vi "Update Test Data Table.vi"(6 "Enum":enum16{"PSU", "Mic"}(ring), 7 "Prev Result in":bool, 8 "Error In":errorcluster, 9 "Test Data In":dbl[](array[numeric]), 10 "Limit In":T1, 11 "Test Data ref in":refnum<vi>) -> (0 "Error Out":errorcluster, 2 "Latest Result Out":bool)   [LabVIEW 2018]
uses:
  Types/LimitType.ctl
panel:
  # "Add PSU Data"
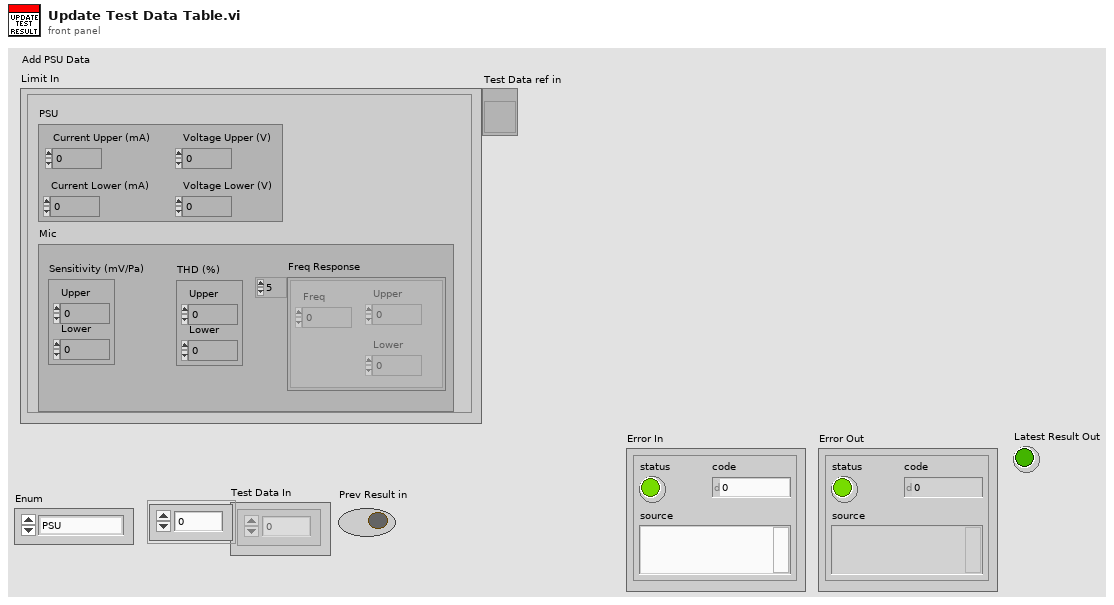
[diagram p1: front panel]
types:
  T1 = typedef "LimitType.ctl" = cluster{"PSU":cluster{"Current Lower (mA)":dbl, "Current Upper (mA)":dbl, "Voltage Lower (V)":dbl, "Voltage Upper (V)":dbl}, "Mic":cluster{"Sensitivity (mV/Pa)":cluster{"Lower":dbl, "Upper":dbl}, "THD (%)":cluster{"Lower":dbl, "Upper":dbl}, "Freq Response":cluster{"Freq":dbl, "Upper":dbl, "Lower":dbl}[]}}
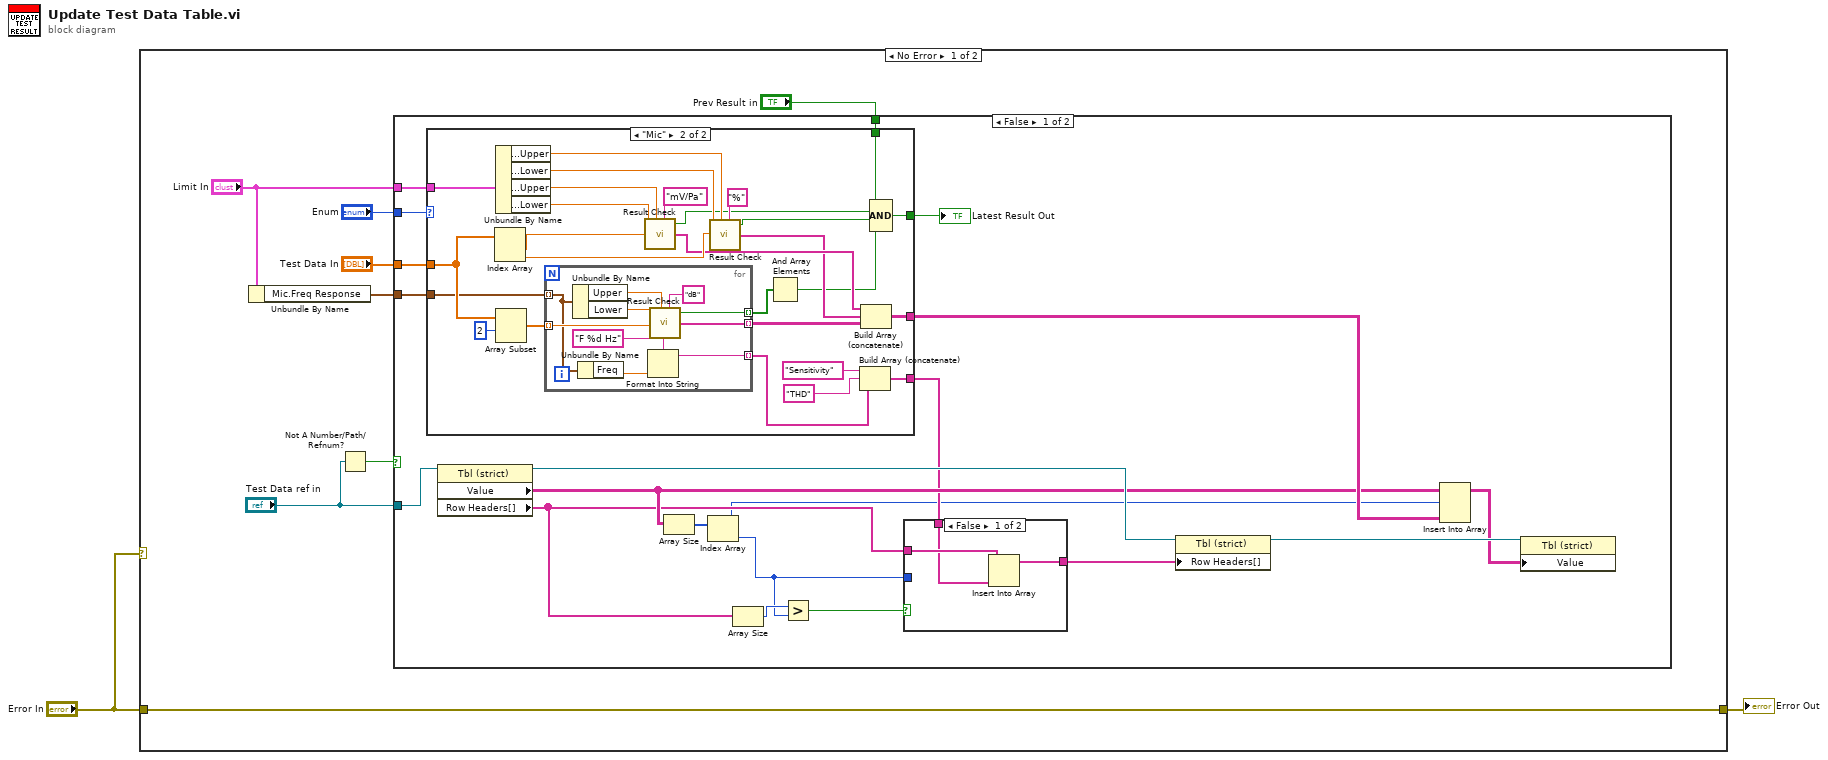
[diagram p0: block diagram]
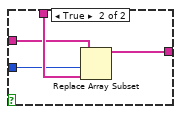
[diagram p2: hidden frame]
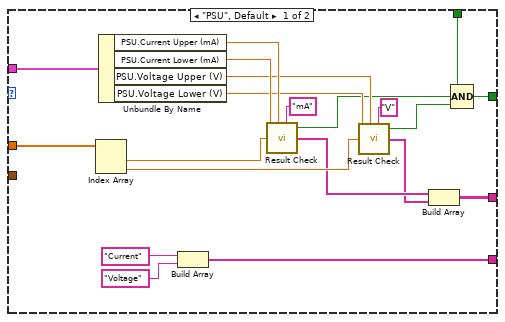
[diagram p3: hidden frame]
diagram:
  n1 = case shown="No Error" "Error In" {
    tunnel: "Error In" -> [w3 w94]
    tunnel: [w3 w94] -> w1
    frame No Error {
      n2 = Unbundle By Name("Limit In") -> ("Mic.Freq Response"=w5:cluster{"Freq":dbl, "Upper":dbl, "Lower":dbl}[])
      n3 = Not A Number/Path/Refnum?(number/path/refnum="Test Data ref in") -> (NaN/Path/Refnum?=w10:bool)
      n4 = case shown="False" w10 {
        tunnel: "Test Data ref in" -> [w29 _]
        tunnel: "Enum" -> [w27 _]
        tunnel: "Limit In" -> [w26 _]
        tunnel: "Test Data In" -> [w25 _]
        tunnel: w5 -> [w17 _]
        tunnel: "Prev Result in" -> [w16 _]
        frame False {
          n5 = case shown="\"Mic\"" w27 {
            tunnel: w26 -> [w56 w83]
            tunnel: w25 -> [w53 w72]
            tunnel: [w46 w63] -> w24
            tunnel: [w41 w67] -> w19
            tunnel: w17 -> [_ w70]
            tunnel: w16 -> [w40 w62]
            tunnel: [w37 w60] -> w15
            frame "PSU", Default {
              n6 = Index Array(array=w53) -> (element #1=w52:dbl, element #2=w49:dbl)  [unwired: 2 in]
              n7 = Unbundle By Name(w56) -> ("PSU.Current Upper (mA)"=w55:dbl, "PSU.Current Lower (mA)"=w54:dbl, "PSU.Voltage Upper (V)"=w51:dbl, "PSU.Voltage Lower (V)"=w50:dbl)
              n8 = Build Array("Current", "Voltage") -> (w41:string[])
              n9 = call "Result Check.vi"("Lower"=w54, "Upper"=w55, "Test Data"=w52, "Unit"="mA") -> ("Result"=w39:bool, "Result String Array Out"=w48:string[])  [unwired: 4 in]
              n10 = call "Result Check.vi"("Lower"=w50, "Upper"=w51, "Test Data"=w49, "Unit"="V") -> ("Result"=w38:bool, "Result String Array Out"=w47:string[])  [unwired: 4 in]
              n11 = Build Array(w48, w47) -> (w46:string[][])
              n12 = Compound Arithmetic op=AND(w40, w39, w38) -> (w37:bool)
            }
            frame "Mic" {
              n13 = Index Array(array=w72) -> (element #1=w77:dbl, element #2=w73:dbl)  [unwired: 2 in]
              n14 = Unbundle By Name(w83) -> ("Mic.THD (%).Upper"=w76:dbl, "Mic.THD (%).Lower"=w75:dbl, "Mic.Sensitivity (mV/Pa).Upper"=w80:dbl, "Mic.Sensitivity (mV/Pa).Lower"=w79:dbl)
              n15 = Array Subset(array=w72, index=2) -> (w69:dbl[])  [unwired: 1 in]
              n16 = for {
                tunnel: w70 -> [w88] mode=indexing
                tunnel: w69 -> [w91] mode=indexing
                tunnel: [w89] -> w64 mode=indexing
                tunnel: [w85] -> w68 mode=indexing
                tunnel: [w84] -> w58 mode=indexing
                n17 = Unbundle By Name(w88) -> ("Upper"=w93:dbl, "Lower"=w92:dbl)
                n18 = Unbundle By Name(w88) -> ("Freq"=w86:dbl)
                n19 = Format Into String(format string="F %d Hz", w86) -> (resulting string=w85:string)  [unwired: 2 in, 1 out]
                n20 = call "Result Check.vi"("Lower"=w92, "Upper"=w93, "Test Data"=w91, "Unit"="dB") -> ("Result"=w84:bool, "Result String Array Out"=w89:string[])  [unwired: 4 in]
              }
              n21 = call "Result Check.vi"("Lower"=w79, "Upper"=w80, "Test Data"=w77, "Unit"="mV/Pa") -> ("Result"=w61:bool, "Result String Array Out"=w66:string[])  [unwired: 4 in]
              n22 = call "Result Check.vi"("Lower"=w75, "Upper"=w76, "Test Data"=w73, "Unit"="%") -> ("Result"=w59:bool, "Result String Array Out"=w65:string[])  [unwired: 4 in]
              n23 = And Array Elements(Boolean array=w58) -> (logical AND=w57:bool)
              n24 = Build Array (concatenate)("Sensitivity", "THD", w68) -> (w67:string[])
              n25 = Build Array (concatenate)(w66, w65, w64) -> (w63:string[][])
              n26 = Compound Arithmetic op=AND(w62, w61, w59, w57) -> (w60:bool)
            }
          }
          "Latest Result Out" <- w15
          n27 = property class="Tbl (strict)"(reference=w29) -> (reference out=w28:refnum<vi>, "Value"=w20:string[][], "Row Headers[]"=w14:string[])  [unwired: 1 in, 1 out]
          n28 = Array Size(array=w20) -> (size(s)=w21:i32[])
          n29 = Index Array(array=w21) -> (element=w11:i32)  [unwired: 1 in]
          n30 = Array Size(array=w14) -> (size(s)=w12:i32)
          n31 = Greater?(x=w12, y=w11) -> (0:w13:bool)
          n32 = case shown="False" w13 {
            tunnel: w19 -> [w31 w36]
            tunnel: [w30 w35] -> w18
            tunnel: w14 -> [w32 w33]
            tunnel: w11 -> [_ w34]
            frame False {
              n33 = Insert Into Array(array=w32, new element=w31) -> (w30:string[])  [unwired: 1 in]
            }
            frame True {
              n34 = Replace Array Subset(array=w33, new element=w36, index=w34) -> (w35:string[])
            }
          }
          n35 = property class="Tbl (strict)"(reference=w28, "Row Headers[]"=w18) -> (reference out=w23:refnum<vi>)  [unwired: 1 in, 1 out]
          n36 = Insert Into Array(array=w20, index (row)=w11, new element=w24) -> (w22:string[][])  [unwired: 1 in]
          n37 = property class="Tbl (strict)"(reference=w23, "Value"=w22) -> ()  [unwired: 1 in, 2 out]
        }
        frame True {
        }
      }
    }
    frame Error {
    }
  }
  "Error Out" <- w1
